vi "posProcessamento.vi"() -> ()   [LabVIEW 2019]
uses:
  <vilib>/Analysis/baseanly.llb/Mean (DBL).vi
  <vilib>/Utility/file.llb/Read Delimited Spreadsheet (DBL).vi
  <vilib>/Utility/file.llb/Read Delimited Spreadsheet (string).vi
  <vilib>/Utility/file.llb/Write Delimited Spreadsheet (string).vi
  <vilib>/Utility/file.llb/Write Delimited Spreadsheet (DBL).vi
  <vilib>/Analysis/NI_AALBase.lvlib
panel:
  in  "Fechar após concluido ?":bool=TRUE
  out "file":string
  out "filenames":string[](array[string])
  out "output":dbl[][](array[numeric])
  out "all rows":dbl[][](array[numeric])
  out "Status":string
  out "Slide":u8(slide) scale=0.0..100.0
  # "Processando"
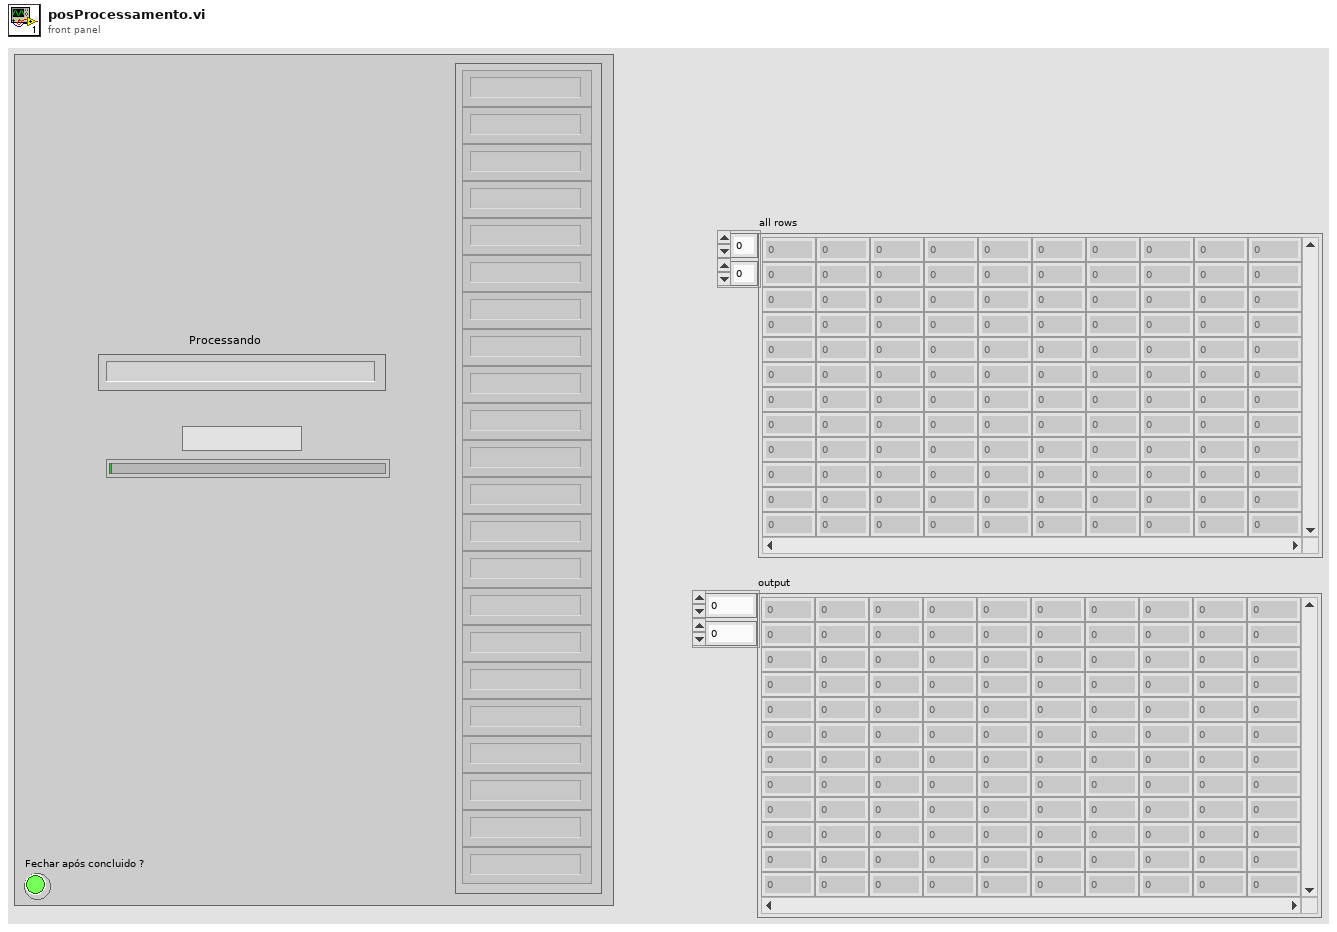
[diagram p1: front panel]
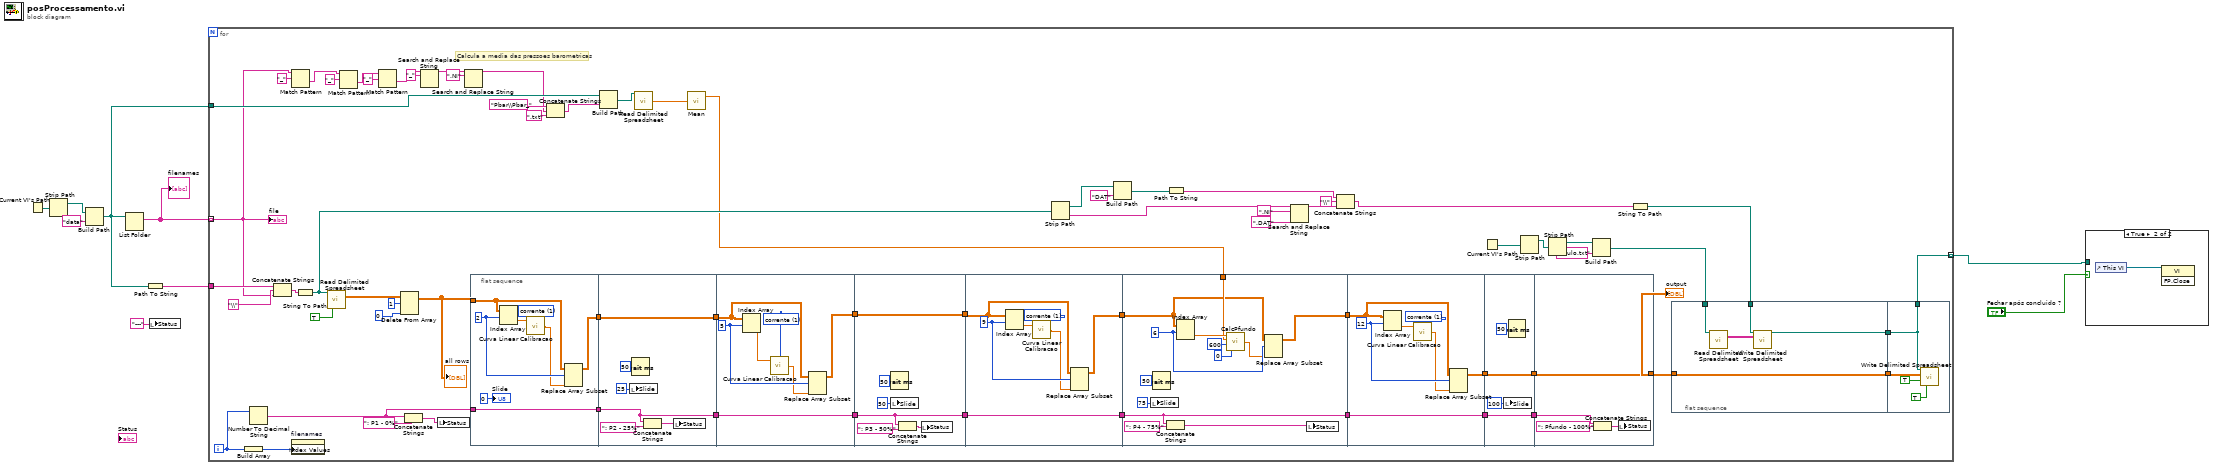
[diagram p0: block diagram]
diagram:
  n1 = Current VI's Path() -> (path=w7:path)
  n2 = Strip Path(path=w7) -> (stripped path=w8:path)  [unwired: 1 out]
  n3 = Build Path(base path=w8, name or relative path="data") -> (appended path=w1:path)
  n4 = List Folder(path=w1) -> (filenames=w6:string[])  [unwired: 3 in, 3 out]
  "filenames" <- w6
  n5 = Path To String(path=w1) -> (string=w5:string)
  n6 = local write "Status"("---" ("Status")) -> ()
  n7 = for {
    tunnel: w6 -> [w11] mode=indexing
    tunnel: w5 -> [w64]
    tunnel: [w15] -> w2 mode=indexing
    tunnel: w1 -> [w24]
    i -> [w47]
    # "Calcula a media das pressoes barometricas"
    n8 = Build Array(w47) -> (w46:i32[])
    n9 = Number To Decimal String(number=w47) -> (decimal integer string=w59:string)  [unwired: 1 in]
    n10 = Concatenate Strings(w64, "\\" ("string"), w11) -> (w51:string)
    n11 = property on="filenames" class="Arr (strict)"("Index Values"=w46) -> ()  [unwired: 2 in, 2 out]
    n12 = Match Pattern(string=w11, regular expression="_") -> (after substring=w10:string)  [unwired: 1 in, 3 out]
    n13 = String To Path(string=w51) -> (path=w45:path)
    n14 = call-poly <vilib>:"Read Delimited Spreadsheet.vi"("file path (dialog if empty)"=w45, "transpose? (F)"=TRUE) -> ("all rows"=w68:dbl[][])  [unwired: 8 in, 5 out]
    n15 = Match Pattern(string=w10, regular expression="_") -> (after substring=w29:string)  [unwired: 1 in, 3 out]
    n16 = Match Pattern(string=w29, regular expression="_") -> (after substring=w28:string)  [unwired: 1 in, 3 out]
    n17 = Delete From Array(array=w68, length=1, index (col)=0 ("disabled index (col)")) -> (array with subset deleted=w65:dbl[][])  [unwired: 1 in, 1 out]
    "all rows" <- w65
    n18 = Concatenate Strings(w59, ": P1 - 0%" ("Status")) -> (w62:string)
    n19 = Search and Replace String(input string=w28, search string="_") -> (result string=w25:string)  [unwired: 6 in, 3 out]
    n20 = local write "Status"(w62) -> ()
    n21 = Search and Replace String(input string=w25, search string=".NI") -> (result string=w21:string)  [unwired: 6 in, 3 out]
    n22 = flat-sequence {
      tunnel: w65 -> [w92]
      tunnel: [w93] -> w77
      tunnel: [w90] -> w60
      tunnel: w59 -> [w90]
      tunnel: w77 -> [w100]
      tunnel: [w100] -> w76
      tunnel: w60 -> [w95]
      tunnel: [w95] -> w58
      tunnel: w76 -> [w106]
      tunnel: [w105] -> w75
      tunnel: w58 -> [w104]
      tunnel: [w104] -> w57
      tunnel: w75 -> [w113]
      tunnel: [w113] -> w74
      tunnel: w57 -> [w108]
      tunnel: [w108] -> w56
      tunnel: w74 -> [w119]
      tunnel: [w118] -> w73
      tunnel: w56 -> [w117]
      tunnel: [w117] -> w55
      tunnel: w73 -> [w123]
      tunnel: [w122] -> w72
      tunnel: w55 -> [w129]
      tunnel: [w129] -> w54
      tunnel: w17 -> [w127]
      tunnel: w72 -> [w138]
      tunnel: [w139] -> w71
      tunnel: w54 -> [w137]
      tunnel: [w137] -> w53
      tunnel: w71 -> [w144]
      tunnel: [w144] -> w70
      tunnel: w53 -> [w141]
      tunnel: [w141] -> w52
      tunnel: [w148] -> w48
      tunnel: w70 -> [w148]
      tunnel: w52 -> [w145]
      frame #0 {
        w87 = u16 1 items=["tensao", "corrente"] ("input type")
        w94 = 2 ("disabled index (col)")
        n23 = Index Array(array=w92, index (row)=w94) -> (element=w89:dbl[])  [unwired: 1 in]
        n24 = call "Curva Linear Calibracao.vi"("input type"=w87, "input"=w89) -> ("output"=w88:dbl[])  [unwired: 2 in]
        n25 = Replace Array Subset(array=w92, new element=w88, index (row)=w94) -> (w93:dbl[][])  [unwired: 1 in]
        "Slide" <- u8 0 ("Slide")
      }
      frame #1 {
        n26 = local write "Slide"(u8 25 ("Slide")) -> ()
        n27 = Wait (ms)(milliseconds to wait=u32 50) -> ()  [unwired: 1 out]
        n28 = Concatenate Strings(w95, ": P2 - 25%" ("Status")) -> (w96:string)
        n29 = local write "Status"(w96) -> ()
      }
      frame #2 {
        w103 = u16 1 items=["tensao", "corrente"] ("input type")
        w107 = 5 ("disabled index (col)")
        n30 = Index Array(array=w106, index (row)=w107) -> (element=w102:dbl[])  [unwired: 1 in]
        n31 = call "Curva Linear Calibracao.vi"("input type"=w103, "input"=w102) -> ("output"=w101:dbl[])  [unwired: 2 in]
        n32 = Replace Array Subset(array=w106, new element=w101, index (row)=w107) -> (w105:dbl[][])  [unwired: 1 in]
      }
      frame #3 {
        n33 = Wait (ms)(milliseconds to wait=u32 50) -> ()  [unwired: 1 out]
        n34 = local write "Slide"(u8 50 ("Slide")) -> ()
        n35 = Concatenate Strings(w108, ": P3 - 50%" ("Status")) -> (w109:string)
        n36 = local write "Status"(w109) -> ()
      }
      frame #4 {
        w116 = u16 1 items=["tensao", "corrente"] ("input type")
        w120 = 9 ("disabled index (col)")
        n37 = Index Array(array=w119, index (row)=w120) -> (element=w115:dbl[])  [unwired: 1 in]
        n38 = call "Curva Linear Calibracao.vi"("input type"=w116, "input"=w115) -> ("output"=w114:dbl[])  [unwired: 2 in]
        n39 = Replace Array Subset(array=w119, new element=w114, index (row)=w120) -> (w118:dbl[][])  [unwired: 1 in]
      }
      frame #5 {
        w124 = 6 ("index (row)")
        n40 = local write "Slide"(u8 75 ("Slide")) -> ()
        n41 = Wait (ms)(milliseconds to wait=u32 50) -> ()  [unwired: 1 out]
        n42 = Concatenate Strings(w129, ": P4 - 75%" ("Status")) -> (w130:string)
        n43 = Index Array(array=w123, index (row)=w124) -> (element=w128:dbl[])  [unwired: 1 in]
        n44 = call "CalcPfundo.vi"("MIN"=0, "MAX"=600, "Pbar"=w127, "input"=w128) -> ("output"=w121:dbl[])
        n45 = Replace Array Subset(array=w123, new element=w121, index (row)=w124) -> (w122:dbl[][])  [unwired: 1 in]
        n46 = local write "Status"(w130) -> ()
      }
      frame #6 {
        w136 = u16 1 items=["tensao", "corrente"] ("input type")
        w140 = 12 ("disabled index (col)")
        n47 = Index Array(array=w138, index (row)=w140) -> (element=w135:dbl[])  [unwired: 1 in]
        n48 = call "Curva Linear Calibracao.vi"("input type"=w136, "input"=w135) -> ("output"=w134:dbl[])  [unwired: 2 in]
        n49 = Replace Array Subset(array=w138, new element=w134, index (row)=w140) -> (w139:dbl[][])  [unwired: 1 in]
      }
      frame #7 {
        n50 = local write "Slide"(u8 100 ("Slide")) -> ()
        n51 = Wait (ms)(milliseconds to wait=u32 50) -> ()  [unwired: 1 out]
      }
      frame #8 {
        n52 = Concatenate Strings(w145, ": Pfundo - 100%" ("Status")) -> (w146:string)
        n53 = local write "Status"(w146) -> ()
      }
    }
    n54 = Concatenate Strings("Pbar\\Pbar_" ("name or relative path"), w21, ".txt" ("string")) -> (w19:string)
    n55 = Build Path(base path=w24, name or relative path=w19) -> (appended path=w20:path)
    n56 = call-poly <vilib>:"Read Delimited Spreadsheet.vi"("file path (dialog if empty)"=w20) -> ("first row"=w18:dbl[])  [unwired: 9 in, 5 out]
    n57 = call-poly <vilib>:"Mean.vi"("X"=w18) -> ("mean"=w17:dbl)  [unwired: 1 out]
    n58 = Strip Path(path=w45) -> (stripped path=w44:path, name=w42:string)
    n59 = Build Path(base path=w44, name or relative path="DAT") -> (appended path=w40:path)
    n60 = Path To String(path=w40) -> (string=w38:string)
    n61 = Search and Replace String(input string=w42, search string=".NI", replace string=".DAT" ("replace string (\"\")")) -> (result string=w41:string)  [unwired: 5 in, 3 out]
    n62 = Concatenate Strings(w38, "\\" ("string"), w41) -> (w39:string)
    n63 = Current VI's Path() -> (path=w35:path)
    n64 = Strip Path(path=w35) -> (stripped path=w33:path)  [unwired: 1 out]
    n65 = Strip Path(path=w33) -> (stripped path=w36:path)  [unwired: 1 out]
    n66 = Build Path(base path=w36, name or relative path="titulo.txt") -> (appended path=w32:path)
    n67 = String To Path(string=w39) -> (path=w16:path)
    n68 = flat-sequence {
      tunnel: w48 -> [w78]
      tunnel: w32 -> [w82]
      tunnel: w16 -> [w80]
      tunnel: [w79] -> w14
      tunnel: [w78] -> w13
      tunnel: [w84] -> w15
      tunnel: w14 -> [w84]
      tunnel: w13 -> [w83]
      frame #0 {
        n69 = call-poly <vilib>:"Read Delimited Spreadsheet.vi"("file path (dialog if empty)"=w82) -> ("all rows"=w81:string[][])  [unwired: 9 in, 5 out]
        n70 = call-poly <vilib>:"Write Delimited Spreadsheet.vi"("file path (dialog if empty)"=w80, "2D data"=w81) -> ("new file path (Not A Path if cancelled)"=w79:path)  [unwired: 12 in, 1 out]
      }
      frame #1 {
        n71 = call-poly <vilib>:"Write Delimited Spreadsheet.vi"("file path (dialog if empty)"=w84, "2D data"=w83, "append to file? (new file:F)"=TRUE, "transpose? (no:F)"=TRUE) -> ()  [unwired: 10 in, 2 out]
      }
    }
    "output" <- w48
    "file" <- w11
  }
  n72 = case shown="True" "Fechar após concluido ?" {
    tunnel: w2 -> [_ _]
    frame False {
    }
    frame True {
      n73 = control-ref of="This VI"() -> (w149:refnum<vi>)
      n74 = invoke class="VI" method="FP.Close"(reference=w149) -> ()  [unwired: 2 in, 3 out]
    }
  }
